vi "Initialize.vi"(8 "error in (no error)":errorcluster, 10 "Name":string, 11 "Filter Wheel in":refnum<class "Filter Wheel.lvclass">) -> (0 "error out":errorcluster, 3 "Filter Wheel out":refnum<class "Filter Wheel.lvclass">)   [LabVIEW 2021, in "Filter Wheel.lvclass"]
uses:
  Filter Wheel Object/Filter Wheel.lvclass
  Filter Wheel Object/Filter Wheel.lvclass/Filter Wheel.ctl
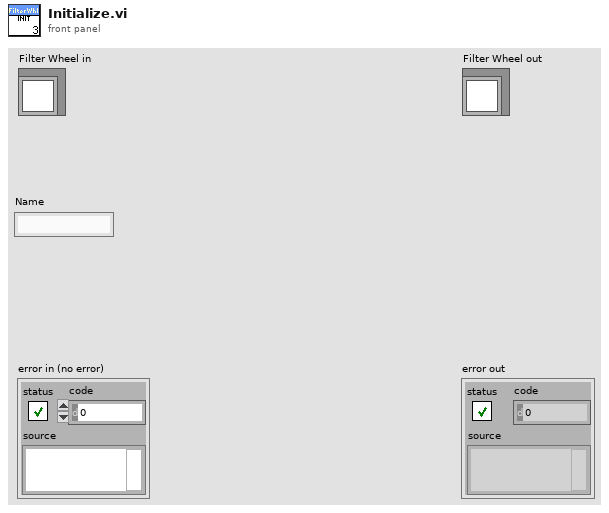
[diagram p1: front panel]
types:
  T1 = typedef "Filter Wheel.lvclass/Filter Wheel configuration.ctl" = cluster{"Num Wheels":i32, "Filters":T2[], "Invalid Combinations":i32[][], "Addr":refnum<visa-resource-name>, "Name":string, "Simulate":bool, "Homing Parameters":T3, "Default Speed":u16}
  T2 = typedef "Filter Wheel.lvclass/Filter Wheel Details.ctl" = cluster{"Names":string[], "Relative Position":i32[], "Wheel Name":string}
  T3 = typedef "Filter Wheel Arduino Homing cluster.ctl" = cluster{"Direction (F: CW)":bool, "Speed":i32, "Accel":i32, "Min Distance":i32, "Short Leg":i32, "Error Cnts":i32}
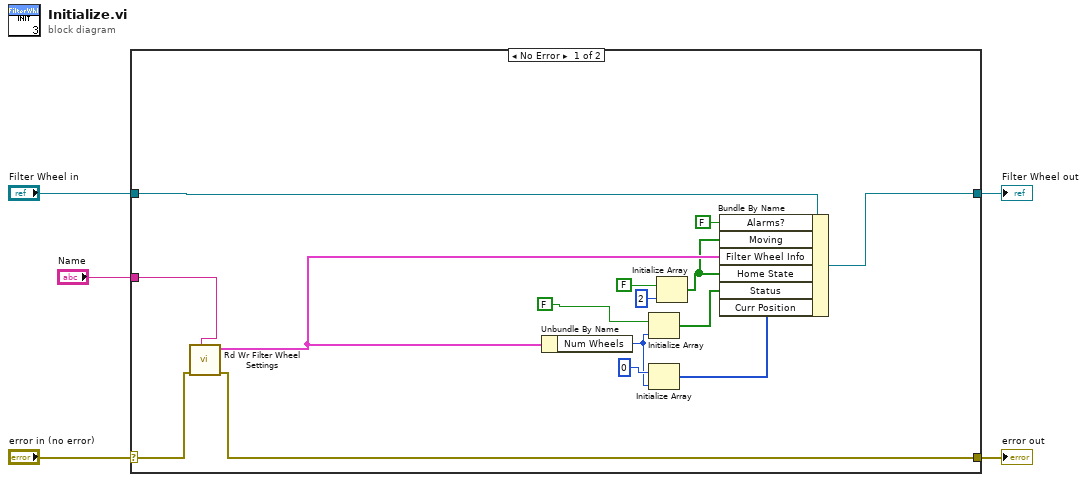
[diagram p0: block diagram]
diagram:
  n1 = case shown="No Error" "error in (no error)" {
    selector: "error in (no error)" -> [w20 w22]
    tunnel: [w19 w22] -> w4
    tunnel: [w14 w21] -> w2
    tunnel: "Filter Wheel in" -> [w11 w21]
    tunnel: "Name" -> [w8 _]
    frame No Error {
      n2 = call "Rd Wr Filter Wheel Settings.vi"("Wheel Name"=w8, "error in (no error)"=w20) -> ("error out"=w19:errorcluster, "Filter Wheel Settings"=w15:T1)  [unwired: 8 in]
      n3 = Unbundle By Name(w15) -> ("Num Wheels"=w13:i32)
      n4 = Initialize Array(FALSE, w13) -> (w18:bool[])
      n5 = Initialize Array(0 ("Numeric"), w13) -> (w16:i32[])
      n6 = Initialize Array(FALSE, 2 ("dimension size")) -> (w7:bool[])
      n7 = Bundle By Name(cluster=w11, "Alarms?"=FALSE, "Moving"=w7, "Filter Wheel Info"=w15, "Home State"=w7, "Status"=w18, "Curr Position"=w16) -> (w14:refnum<class "Filter Wheel.lvclass">)
    }
    frame Error {
    }
  }
  "error out" <- w4
  "Filter Wheel out" <- w2
